vi "CSM-Logger-Thread.vi"(4 "Log Limit":T1={"file size (in bytes)"=10000000, "file num"=2} {"file size (in bytes)" format="%.0p"}, 6 "Exit When All Module Exist? (F)":bool, 7 "Format String":string="%<%Y/%m/%d %H:%M:%S%3u>T", 8 "error in (no error)":errorcluster, 9 "WatchDogQ":refnum<queue>, 10 "GlobalLogFilter.lvclass":refnum<class "LogFilter.lvclass">, 11 "File Path (Use Dialog)":path) -> (0 "error out":errorcluster)   [LabVIEW 2017, in "CSM File Logger.lvlib"]
doc: "#### CSM-Logger-Thread.vi\n\nStarts the CSM Global Log file logging thread VI.\n\n> [!NOTE] Principle of CSM File Logger\n> By subscribing to the CSM's Global Log Event, all CSM activity information in the application can be recorded for later analysis and error localization.\n> The file is a text file with the extension .csmlog, which can be opened with Notepad or other text editing tools.\n\n\n-- <b>Controls</b> --\n- <b>Log File Path</b>: Path to the log file\n- <b>log limit</b>: Log file limit\n- <b>Timestamp format</b>: Timestamp format\n- <b>WatchDogQ</b>: WatchDog resource for detecting if the main program has exited\n- <b>GlobalLogFilter.lvclass</b>: Event filter object\n- <b>Exit When All Module Exist?(F)</b>: Exit after all CSM modules exit or not"
uses:
  CSM File Logger.lvlib
  CSM File Logger Limit.ctl
  _Support/GlobalEvent/LogFilter/LogFilter.lvclass
  _Support/Typedef/_CSM_List Module Scope.ctl
  Communicable State Machine.lvlib
  _Shared/CSM Shared.lvlib
panel:
  in  "internal Stop":bool
  out "#MsgInQueue":i32
  out "size (in bytes)":i64
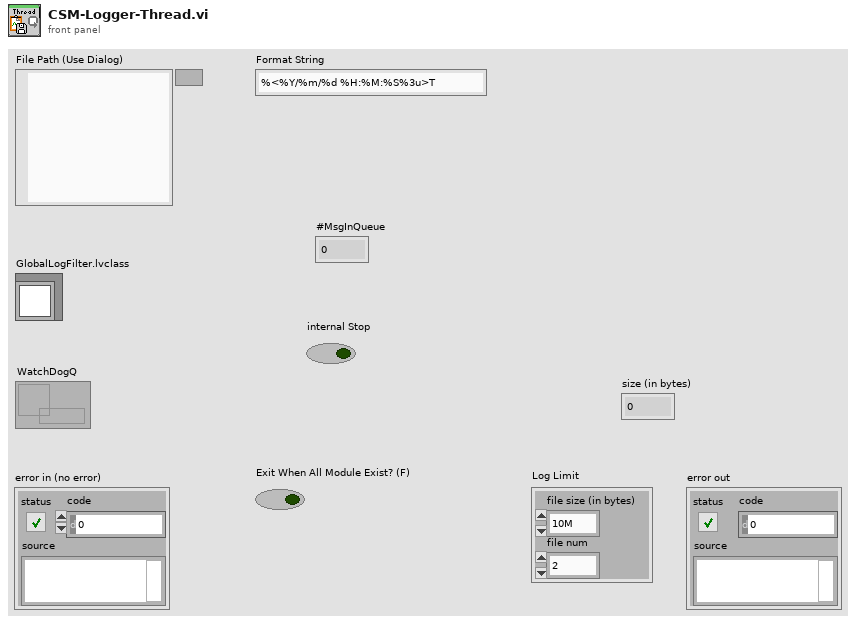
[diagram p1: front panel]
types:
  T1 = typedef "CSM File Logger.lvlib/CSM File Logger Limit.ctl" = cluster{"file size (in bytes)":i64, "file num":i32}
  T2 = typedef "Communicable State Machine.lvlib/_CSM_GlobalLog_MSG_TYPE.ctl" = enum16{"User Log", "State Change", "Status", "Interrupt", "Register", "Unregister", "Error Log", "Module Created", "Module Destroyed"}
  T3 = typedef "Communicable State Machine.lvlib/_CSM_GlobalLog_STATE_TYPE.ctl" = enum16{"State - Internal State", "State - External Message", "State - Response", "State - Complete"}
  T4 = cluster{"Global":cluster{"CSM":string[], "LogType":T2[], "State":string[], "StateType":T3[]}, "CSM":cluster{"LogType":cluster{"CSM":string, "LogType":T2}[], "State":cluster{"CSM":string, "State":string}[], "StateType":cluster{"CSM":string, "LogType":T3}[]}, "PeriodicLog":cluster{"Enable":bool, "Threshold(#/s)":dbl, "CheckPeriod(s)":dbl}}
  T5 = cluster{"Queue":path[], "folder":path, "name":string, "index":i32, "Log Limit":T1}
  T6 = enum16{"open", "replace", "create", "open or create", "replace or create", "replace or create with confirmation"}
  T7 = typedef "Communicable State Machine.lvlib/_CSM_List Module Scope.ctl" = enum16{"Normal", "System Only", "All"}
  T8 = typedef "Communicable State Machine.lvlib/Periodic String Filter Level.ctl" = enum16{"normal", "L1", "L2", "L3", "L4"}
  T9 = typedef "Communicable State Machine.lvlib/_CSM_GlobalLog_MSG.ctl" = cluster{"Name (\"\" to Use UUID)":string, "Current State":string, "Arguments":string, "Source Message":T10, "Source Module":string, "Complete(T)/Start(F)":bool, "LogType":T2, "Time Stamp":timestamp}
  T10 = typedef "Communicable State Machine.lvlib/_CSM_Response Source Message.ctl" = cluster{"‘State":string, "’Arguments":string, "’Error":errorcluster}
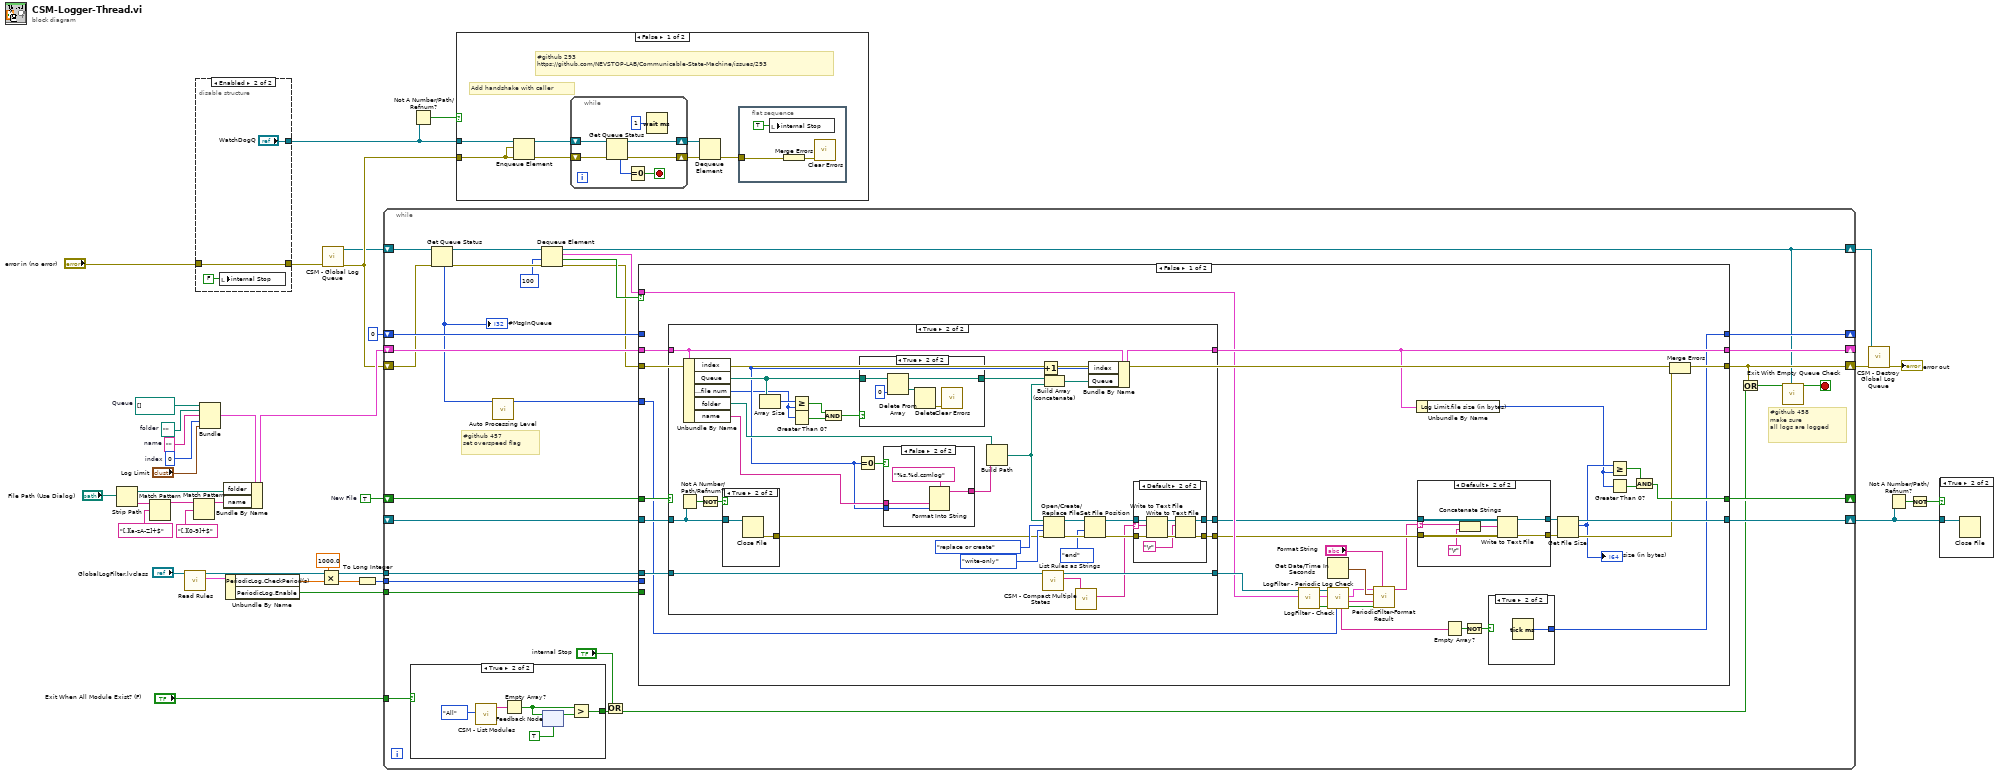
[diagram p0: block diagram]
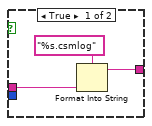
[diagram p6: hidden frame]
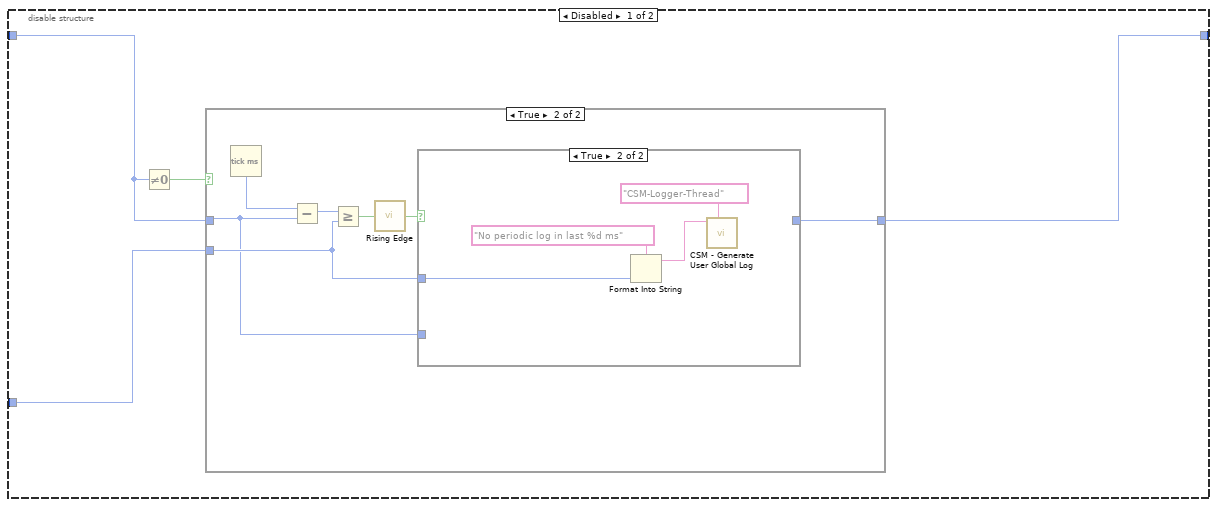
[diagram p10: hidden frame]
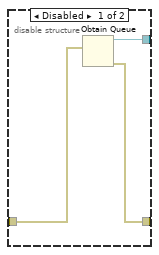
[diagram p15: hidden frame]
diagram:
  w24 = ""  # name
  w27 = 0  # index
  w28 = path ""  # folder
  w29 = path[] []  # Queue
  w30 = TRUE  # New File
  n1 = Strip Path(path="File Path (Use Dialog)") -> (stripped path=w17:path, name=w23:string)
  n2 = Match Pattern(string=w23, regular expression="[.][a-zA-Z]+$") -> (before substring=w20:string)  [unwired: 1 in, 3 out]
  n3 = call "Read Rules.vi"("LogFilter In"="GlobalLogFilter.lvclass") -> ("Rules"=w12:T4, "LogFilter Out"=w13:refnum<class "LogFilter.lvclass">)  [unwired: 8 in, 1 out]
  n4 = Match Pattern(string=w20, regular expression="[.][0-9]+$") -> (before substring=w18:string)  [unwired: 1 in, 3 out]
  n5 = disable-structure shown="Enabled" {
    disable-tunnel: [w38 "WatchDogQ"] -> w36
    disable-tunnel: [w40 w42] -> w1
    disable-tunnel: "error in (no error)" -> [w39 w42]
    frame Disabled {
      n6 = Obtain Queue(element data type=w39) -> (queue out=w38:refnum<queue>, error out=w40:errorcluster)  [unwired: 4 in, 1 out]
    }
    frame Enabled {
      n7 = local write "internal Stop"(FALSE ("internal Stop")) -> ()
    }
  }
  n8 = Bundle("Queue"=w29, "folder"=w28, "name"=w24, "index"=w27, "Log Limit"="Log Limit") -> (w25:T5)  [unwired: 1 in]
  n9 = Bundle By Name(cluster=w25, "folder"=w17, "name"=w18) -> (w19:T5)
  n10 = Unbundle By Name(w12) -> ("PeriodicLog.CheckPeriod(s)"=w10:dbl, "PeriodicLog.Enable"=w11:bool)
  n11 = Multiply(x=1000.0, y=w10) -> (x*y=w9:dbl)
  n12 = call "CSM - Global Log Queue.vi"("Error In"=w1) -> ("error out"=w5:errorcluster, "GlobalEvent Queue"=w2:refnum<queue>)  [unwired: 9 in]
  n13 = To Long Integer(number=w9) -> (32bit integer=w7:i32)
  n14 = while {
    shift-right: [w72] -> w37
    shift-left: w5 -> [w55]
    shift-right: [w70] -> w32
    shift-left: _ -> [w71]
    tunnel: "Exit When All Module Exist? (F)" -> [w54]
    shift-right: [w68] -> _
    shift-left: w30 -> [w69]
    shift-right: [w66] -> _
    shift-left: w19 -> [w67]
    tunnel: w13 -> [w65]
    tunnel: w11 -> [w62]
    tunnel: w7 -> [w64]
    shift-right: [w63] -> _
    shift-left: u32 0 ("millisecond timer value") -> [w61]
    shift-right: [w46] -> w4
    shift-left: w2 -> [w58]
    stop <- w47 stop-if-true
    # "#github 458\nmake sure \nall logs are logged"
    # "#github 457\nset overspeed flag"
    n15 = case shown="True" w54 {
      tunnel: [_ w204] -> w53
      frame False {
      }
      frame True {
        n16 = call "CSM - List Modules.vi"("Scope (Normal)"=_CSM_List_Module_Scope."All" ("Mode")) -> ("Module Names"=w208:string[])  [unwired: 9 in, 1 out]
        n17 = Empty Array?(array=w208) -> (empty?=w207:bool)
        n18 = feedback #1(TRUE ("All?")) -> (w206:bool)
        n19 = feedback-in #1(w207) -> ()
        n20 = Greater?(x=w207, y=w206) -> (0:w204:bool)
      }
    }
    n21 = Get Queue Status(queue=w58, error in (no error)=w55) -> (queue out=w57:refnum<queue>, error out=w56:errorcluster, # elements in queue=w45:i32)  [unwired: 1 in, 5 out]
    "#MsgInQueue" <- w45
    n22 = call "Auto Processing Level.vi"("#Left In Q"=w45) -> ("Level"=w44:T8)  [unwired: 8 in, 2 out]
    n23 = Dequeue Element(queue=w57, timeout in ms (-1)=100, error in (no error)=w56) -> (queue out=w46:refnum<queue>, element=w49:T9, timed out?=w60:bool, error out=w59:errorcluster)
    n24 = Or(x="internal Stop", y=w53) -> (x .or. y?=w51:bool)
    n25 = case shown="False" w60 {
      tunnel: w59 -> [w106 w185]
      tunnel: [w105 w185] -> w72
      tunnel: w71 -> [w104 w184]
      tunnel: [w103 w184] -> w70
      tunnel: w69 -> [w102 w183]
      tunnel: [w101 w183] -> w68
      tunnel: w67 -> [w100 w182]
      tunnel: [w99 w182] -> w66
      tunnel: w65 -> [w98 _]
      tunnel: w64 -> [_ w181]
      tunnel: [w97 w179] -> w63
      tunnel: w62 -> [_ _]
      tunnel: w61 -> [_ w180]
      tunnel: w49 -> [w86 _]
      tunnel: w44 -> [w81 _]
      frame False {
        n26 = case shown="True" w102 {
          tunnel: w104 -> [w119 w151]
          tunnel: [_ w123] -> w83
          tunnel: [w119 w124] -> w82
          tunnel: [w118 w140] -> w99
          tunnel: w100 -> [w118 w142]
          tunnel: [w117 w122] -> w91
          tunnel: w98 -> [w117 w127]
          frame False {
          }
          frame True {
            n27 = Not A Number/Path/Refnum?(number/path/refnum=w151) -> (NaN/Path/Refnum?=w152:bool)
            n28 = Unbundle By Name(w142) -> ("index"=w132:i32, "Queue"=w143:path[], "Log Limit.file num"=w129:i32, "folder"=w136:path, "name"=w135:string)
            n29 = Not(x=w152) -> (.not. x?=w153:bool)
            n30 = case shown="True" w153 {
              tunnel: w151 -> [_ w178]
              tunnel: [_ w177] -> w145
              frame False {
              }
              frame True {
                n31 = Close File(refnum=w178) -> (error out=w177:errorcluster)  [unwired: 1 in, 1 out]
              }
            }
            n32 = Array Size(array=w143) -> (size(s)=w144:i32)
            n33 = Greater Or Equal?(x=w144, y=w129) -> (x >= y?=w131:bool)
            n34 = Greater Than 0?(x=w129) -> (x > 0?=w130:bool)
            n35 = And(x=w131, y=w130) -> (x .and. y?=w128:bool)
            n36 = Equal To 0?(x=w132) -> (x = 0?=w133:bool)
            n37 = case shown="True" w128 {
              tunnel: w143 -> [w171 w176]
              tunnel: [w171 w172] -> w141
              frame False {
              }
              frame True {
                n38 = Delete From Array(array=w176, index=0) -> (deleted portion=w174:path, array with subset deleted=w172:path[])  [unwired: 1 in]
                n39 = Delete(path (use dialog)=w174) -> (error out=w173:errorcluster)  [unwired: 4 in, 2 out]
                n40 = call <vilib>:"Clear Errors.vi"("error in (no error)"=w173) -> ()  [unwired: 5 in, 2 out]
              }
            }
            n41 = case shown="False" w133 {
              tunnel: [w165 w169] -> w137
              tunnel: w135 -> [w164 w168]
              tunnel: w132 -> [_ w167]
              frame True {
                n42 = Format Into String(format string="%s.csmlog", w164) -> (resulting string=w165:string)  [unwired: 2 in, 1 out]
              }
              frame False {
                n43 = Format Into String(format string="%s.%d.csmlog", w168, w167) -> (resulting string=w169:string)  [unwired: 2 in, 1 out]
              }
            }
            n44 = Build Path(base path=w136, name or relative path=w137) -> (appended path=w134:path)
            n45 = Increment(x=w132) -> (x+1=w138:i32)
            n46 = call "List Rules as Strings.vi"("GlobalLogFilter In"=w127) -> ("Rule Strings"=w121:string[], "GlobalLogFilter Out"=w122:refnum<class "LogFilter.lvclass">)  [unwired: 8 in, 1 out]
            n47 = Open/Create/Replace File(file path (use dialog)=w134, error in=w145, operation (0:open)=T6."replace or create", access (0:read/write)=enum16{"read/write", "read-only", "write-only"}."write-only") -> (refnum out=w150:refnum<file>, error out=w149:errorcluster)  [unwired: 2 in, 1 out]
            n48 = Build Array (concatenate)(w141, w134) -> (w139:path[])
            n49 = call "CSM - Compact Multiple States.vi"("Multiple States"=w121) -> ("States"=w120:string)  [unwired: 9 in]
            n50 = Set File Position(refnum=w150, from (0:start)=enum16{"start", "end", "current"}."end", error in=w149) -> (refnum out=w125:refnum<file>, error out=w126:errorcluster)  [unwired: 1 in]
            n51 = Bundle By Name(cluster=w142, "index"=w138, "Queue"=w139) -> (w140:T5)
            n52 = case shown="Default" w120 {
              selector: w120 -> [_ w163]
              tunnel: w126 -> [w154 w162]
              tunnel: w125 -> [w155 w161]
              tunnel: [w155 w158] -> w124
              tunnel: [w154 w157] -> w123
              frame "" {
              }
              frame Default {
                n53 = Write to Text File(file (use dialog)=w161, text=w163, error in=w162) -> (refnum out=w159:refnum<file>, error out=w160:errorcluster)  [unwired: 1 in, 1 out]
                n54 = Write to Text File(file (use dialog)=w159, text="\r", error in=w160) -> (refnum out=w158:refnum<file>, error out=w157:errorcluster)  [unwired: 1 in, 1 out]
              }
            }
          }
        }
        n55 = call "LogFilter - Check.vi"("Cross CSM Data In"=w86, "GlobalLogFilter In"=w91) -> ("Matched? (Dup)"=w77:bool, "Cross CSM Data Out"=w78:T9, "GlobalLogFilter.lvclass (Dup)"=w79:refnum<class "LogFilter.lvclass">)  [unwired: 7 in]
        n56 = Get Date/Time In Seconds() -> (seconds since 1Jan1904=w80:timestamp)
        n57 = call "LogFilter - Periodic Log Check.vi"("Level (Normal)"=w81, "Matched Previous?"=w77, "Cross CSM Data In"=w78, "GlobalLogFilter In"=w79) -> ("Matched? (Dup)"=w74:bool, "Additional Info"=w75:string[], "Cross CSM Data Out"=w76:T9, "Filtered Status"=w90:string[])  [unwired: 3 in, 1 out]
        n58 = call "PeriodicFilter-Format Result.vi"("Time Format String"="Format String", "Filtered"=w74, "Additional Info"=w75, "Current Time"=w80, "Cross CSM Data In"=w76) -> ("States"=w73:string)  [unwired: 6 in]
        n59 = Unbundle By Name(w99) -> ("Log Limit.file size (in bytes)"=w92:i64)
        n60 = case shown="Default" w73 {
          selector: w73 -> [_ w110]
          tunnel: w83 -> [w107 w115]
          tunnel: w82 -> [w108 w114]
          tunnel: [w108 w113] -> w85
          tunnel: [w107 w112] -> w84
          frame "" {
          }
          frame Default {
            n61 = Concatenate Strings(w110, "\r") -> (w109:string)
            n62 = Write to Text File(file (use dialog)=w114, text=w109, error in=w115) -> (refnum out=w113:refnum<file>, error out=w112:errorcluster)  [unwired: 1 in, 1 out]
          }
        }
        n63 = Empty Array?(array=w90) -> (empty?=w89:bool)
        n64 = Not(x=w89) -> (.not. x?=w88:bool)
        n65 = case shown="True" w88 {
          tunnel: [_ w116] -> w97
          frame False {
          }
          frame True {
            n66 = Tick Count (ms)() -> (millisecond timer value=w116:u32)
          }
        }
        n67 = Get File Size(file=w85, error in=w84) -> (refnum out=w103:refnum<file>, size (in bytes)=w95:i64, 0:w96:errorcluster)
        "size (in bytes)" <- w95
        n68 = Greater Or Equal?(x=w95, y=w92) -> (x >= y?=w94:bool)
        n69 = Greater Than 0?(x=w92) -> (x > 0?=w93:bool)
        n70 = And(x=w94, y=w93) -> (x .and. y?=w101:bool)
        n71 = Merge Errors(w106, w96) -> (w105:errorcluster)
      }
      frame True {
        n72 = disable-structure shown="Enabled" {
          disable-tunnel: w181 -> [w189 _]
          disable-tunnel: w180 -> [w188 _]
          disable-tunnel: [w186 _] -> w179
          frame Disabled {
            n73 = Not Equal To 0?(x=w188) -> (x != 0?=w187:bool)
            n74 = case shown="True" w187 {
              tunnel: w188 -> [w190 w193]
              tunnel: w189 -> [_ w195]
              tunnel: [w190 w194] -> w186
              frame False {
              }
              frame True {
                n75 = Tick Count (ms)() -> (millisecond timer value=w197:u32)
                n76 = Subtract(x=w197, y=w193) -> (x-y=w196:u32)
                n77 = Greater Or Equal?(x=w196, y=w195) -> (x >= y?=w192:bool)
                n78 = call "Rising Edge.vi"("Signal"=w192) -> ("Rising Edge"=w191:bool)
                n79 = case shown="True" w191 {
                  tunnel: w195 -> [_ w199]
                  tunnel: [w198 _] -> w194
                  tunnel: w193 -> [w198 _]
                  frame False {
                  }
                  frame True {
                    n80 = Format Into String(format string="No periodic log in last %d ms" ("Log"), w199) -> (resulting string=w200:string)  [unwired: 2 in, 1 out]
                    n81 = call "CSM - Generate User Global Log.vi"("Place (\"\" to Use VI's Name)"="CSM-Logger-Thread" ("Place(\"\" to use VI's Name)"), "Log"=w200) -> ()  [unwired: 9 in, 1 out]
                  }
                }
              }
            }
          }
          frame Enabled {
          }
        }
      }
    }
    n82 = Or(x=w72, y=w51) -> (x .or. y?=w48:bool)
    n83 = call "Exit With Empty Queue Check.vi"("Queue"=w46, "Stop"=w48) -> ("Exit"=w47:bool)  [unwired: 8 in, 1 out]
  }
  n84 = Not A Number/Path/Refnum?(number/path/refnum=w36) -> (NaN/Path/Refnum?=w35:bool)
  n85 = case shown="False" w35 {
    tunnel: w36 -> [w214 _]
    tunnel: w5 -> [w209 _]
    frame False {
      # "#github 293 \nhttps://github.com/NEVSTOP-LAB/Communicable-State-Machine/issues/293"
      # "Add handshake with caller"
      n86 = Enqueue Element(queue=w214, element=w209, error in (no error)=w209) -> (queue out=w213:refnum<queue>, error out=w211:errorcluster)  [unwired: 1 in, 1 out]
      n87 = while {
        shift-right: [w221] -> w212
        shift-left: w213 -> [w222]
        shift-right: [w219] -> w210
        shift-left: w211 -> [w220]
        stop <- w217 stop-if-true
        n88 = Get Queue Status(queue=w222, error in (no error)=w220) -> (queue out=w221:refnum<queue>, error out=w219:errorcluster, # elements in queue=w218:i32)  [unwired: 1 in, 5 out]
        n89 = Equal To 0?(x=w218) -> (x = 0?=w217:bool)
        n90 = Wait (ms)(milliseconds to wait=u32 1) -> ()  [unwired: 1 out]
      }
      n91 = Dequeue Element(queue=w212, error in (no error)=w210) -> (error out=w215:errorcluster)  [unwired: 1 in, 3 out]
      n92 = flat-sequence {
        tunnel: w215 -> [w225]
        frame #0 {
          n93 = local write "internal Stop"(TRUE ("internal Stop")) -> ()
          n94 = Merge Errors(w225) -> (w224:errorcluster)
          n95 = call <vilib>:"Clear Errors.vi"("error in (no error)"=w224) -> ()  [unwired: 5 in, 2 out]
        }
      }
    }
    frame True {
    }
  }
  n96 = call "CSM - Destroy Global Log Queue.vi"("Error In"=w37, "Global Log Queue"=w4) -> ("error out"=→"error out":errorcluster)  [unwired: 9 in]
  n97 = Not A Number/Path/Refnum?(number/path/refnum=w32) -> (NaN/Path/Refnum?=w33:bool)
  n98 = Not(x=w33) -> (.not. x?=w31:bool)
  n99 = case shown="True" w31 {
    tunnel: w32 -> [_ w226]
    frame False {
    }
    frame True {
      n100 = Close File(refnum=w226) -> ()  [unwired: 1 in, 2 out]
    }
  }
